vi "Drive Mode.vi"(8 "reinitialize? (F)":bool) -> ()   [LabVIEW 2011]
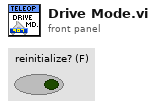
[diagram p1: front panel]
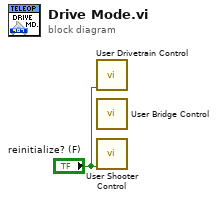
[diagram p0: block diagram]
diagram:
  n1 = call "User Drivetrain Control.vi"("reinitialize"="reinitialize? (F)") -> ()  [unwired: 11 in]
  n2 = call "User Bridge Control.vi"() -> ()  [unwired: 12 in]
  n3 = call "User Shooter Control.vi"("reinitialize? (F)"="reinitialize? (F)") -> ()  [unwired: 11 in]
